vi "Day5_Validation.vi"() -> ()   [LabVIEW 2025]
uses:
  <vilib>/Platform/TimedLoop/XDataNode/timing_clust.ctl
  <vilib>/Platform/TimedLoop/XDataNode/nitl_modes.ctl
  <vilib>/Platform/TimedLoop/XDataNode/wakeup.ctl
  <vilib>/Utility/error.llb/Trim Whitespace One-Sided.vi
  <vilib>/Instr/_visa.llb/VISA Configure Serial Port (Instr).vi
  <vilib>/platform/TimedLoop/XDataNode/XDataNode.xnode
  <vilib>/Platform/TimedLoop/XDataNode/XDNodeRunTimeDep.lvlib
  <vilib>/ptbypt/NI_PtbyPt.lvlib
panel:
  out "Touch FAIL":bool
  out "Touch PASS":bool
  in  "Touch Lo Limit":dbl
  in  "Touch Hi Limit":dbl
  out "Max":dbl
  out "Min":dbl
  out "Mean":dbl
  out "Std Dev":dbl
  out "mean":dbl format="%0.2f"
  out "ADC (mv)":dbl
  out "Touch Pin":dbl
  out "Hall Sensor":dbl
  out "Timestamp":dbl
  in  "stop":bool
  # "Day 4: Statistics engine using a custom SubVI. Collects last 20 Touch Pin readings and computes live stats"
  # "Mean PtByPt: continuous running average since session start"
  # "Stats SubVI outputs: computed from a rolling buffer of the last 20 Touch Pin samples."
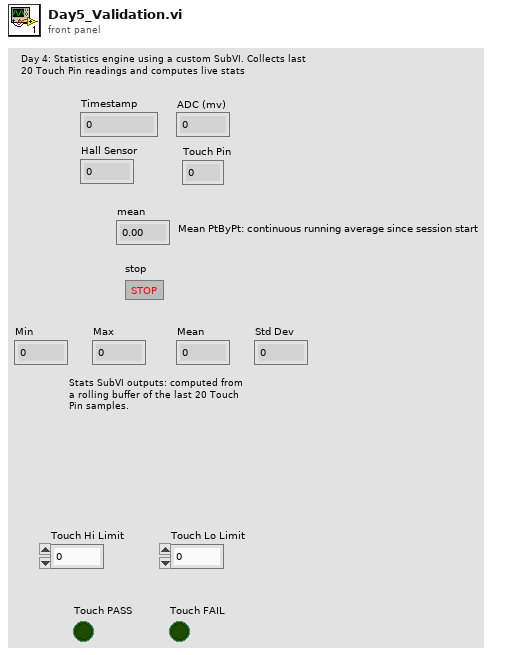
[diagram p1: front panel]
types:
  T1 = typedef "XDNodeRunTimeDep.lvlib/timing_clust.ctl" = cluster{"Expected End [f-1]":u64, "Actual End [f-1]":u64, "Finished Late? [f-1]":bool, "Expected End [i-1]":u64, "Actual End [i-1]":u64, "Finished Late? [i-1]":bool, "Expected Start [i]":u64, "Actual Start [i]":u64, "Expected Start [f]":u64, "Actual Start [f]":u64, "Source Name":string, "Structure Name":string, "Period":i64, "Deadline":i64, "Offset":i64, "Start":i64, "Priority":i32, "Timeout":i32, "Mode":T2, "Wakeup Reason":T3, "Error":errorcluster, "Source Type":string, "Secondary Source Type":string, "Global End Time":u64, "Global Start Time":u64, "Frame Duration":u64, "Iteration Duration":u64, "Assigned CPU":i32, "I/O Scan Engine Mode":u32}
  T2 = typedef "XDNodeRunTimeDep.lvlib/nitl_modes.ctl" = enum32{"No Change", "Process missed periods, maintain original phase", "Discard missed periods, maintain original phase", "Process missed periods, ignore original phase", "Discard missed periods, ignore original phase"}
  T3 = typedef "XDNodeRunTimeDep.lvlib/wakeup.ctl" = enum32{"Normal", "Aborted", "Asynchronous wakeup", "Timing source error", "Timed loop error", "Timeout"}
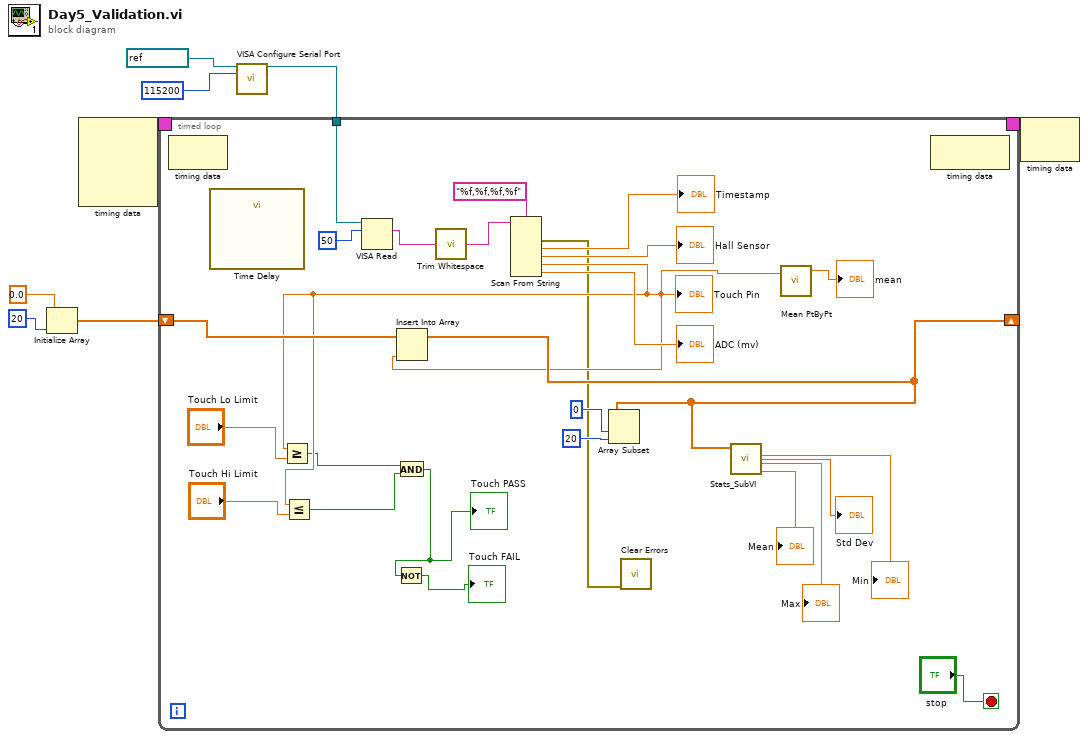
[diagram p0: block diagram]
diagram:
  n1 = Initialize Array "Initialize Array"(0.0 ("element"), 20 ("dimension size")) -> (w3:dbl[])
  n2 = node-c288() -> (w6:T1)  [unwired: 4 in]
  n3 = call-poly "VISA Configure Serial Port"("VISA resource name"=refnum<visa-resource-name> "COM3", "baud rate (9600)"=u32 115200) -> ("VISA resource name out"=w4:refnum<visa-resource-name>)  [unwired: 12 in, 1 out]
  n4 = timed-loop {
    timing: w6 -> [_]
    timing-out: [_] -> w5
    tunnel: w4 -> [w27]
    shift-right: [w21] -> _
    shift-left: w3 -> [w24]
    stop <- "stop" stop-if-true
    n5 = node-c288() -> ()  [unwired: 1 in, 1 out]
    n6 = call "Time Delay"() -> ()  [unwired: 11 in, 1 out]
    n7 = VISA Read(VISA resource name=w27, byte count=u32 50) -> (read buffer=w33:string)  [unwired: 1 in, 3 out]
    n8 = call <vilib>:"Trim Whitespace.vi"("string"=w33) -> ("trimmed string"=w32:string)  [unwired: 1 in]
    n9 = Scan From String "Scan From String"(format string="%f,%f,%f,%f", input string=w32) -> (error out=w11:errorcluster, output 1=→"Timestamp":dbl, output 2=→"Hall Sensor":dbl, output 3=w15:dbl, output 4=→"ADC (mv)":dbl)  [unwired: 6 in, 2 out]
    "Touch Pin" <- w15
    n10 = Greater Or Equal?(x=w15, y="Touch Lo Limit") -> (x >= y?=w14:bool)
    n11 = Less Or Equal?(x=w15, y="Touch Hi Limit") -> (x <= y?=w13:bool)
    n12 = Insert Into Array "Insert Into Array"(array=w24, new element=w15) -> (w21:dbl[])  [unwired: 1 in]
    n13 = And(x=w14, y=w13) -> (x .and. y?=w9:bool)
    "Touch PASS" <- w9
    n14 = Not(x=w9) -> (.not. x?=→"Touch FAIL":bool)
    n15 = Array Subset "Array Subset"(array=w21, index=0, length=20) -> ()  [unwired: 1 out]
    n16 = call <vilib>:"Clear Errors.vi"("error in (no error)"=w11) -> ()  [unwired: 5 in, 2 out]
    n17 = call "Stats_SubVI.vi"("Input Array"=w21) -> ("Std Dev"=→"Std Dev":dbl, "Mean"=→"Mean":dbl, "Max"=→"Max":dbl, "Min"=→"Min":dbl)
    n18 = call <vilib>:"Mean PtByPt.vi"("x"=w15) -> ("mean"=→"mean":dbl)  [unwired: 3 in, 1 out]
    n19 = node-c288() -> ()  [unwired: 1 in, 1 out]
  }
  n20 = node-c288(w5) -> ()  [unwired: 1 out]
